vi "关键参数交互.vi"(9 "量程选择":enum16{"低量程", "高量程", "0-2量程"}(ring), 10 "测量模式(公式)":u16(ring)=1 items=["水样测试"=1, "标样核查"=2, "零点核查"=3, "跨度核查"=4, "空白测试"=5, "平行样"=6, "加标回收"=7], 11 "模型":enum32{"线性", "多项式"}(ring)) -> ()   [LabVIEW 2016]
panel:
  out "x != y?":T1
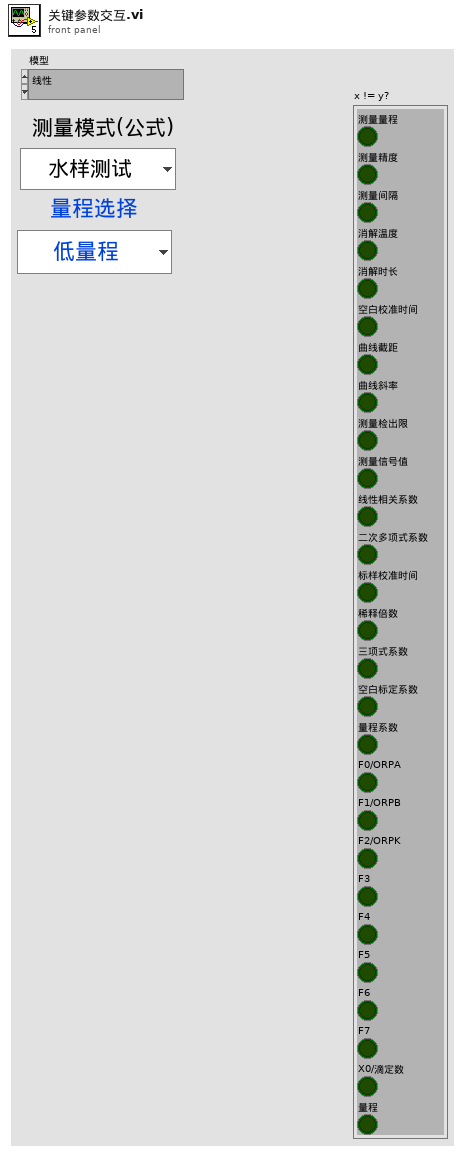
[diagram p1: front panel]
types:
  T1 = cluster{"测量量程":bool, "测量精度":bool, "测量间隔":bool, "消解温度":bool, "消解时长":bool, "空白校准时间":bool, "曲线截距":bool, "曲线斜率":bool, "测量检出限":bool, "测量信号值":bool, "线性相关系数":bool, "二次多项式系数":bool, "标样校准时间":bool, "稀释倍数":bool, "三项式系数":bool, "空白标定系数":bool, "量程系数":bool, "F0/ORPA":bool, "F1/ORPB":bool, "F2/ORPK":bool, "F3":bool, "F4":bool, "F5":bool, "F6":bool, "F7":bool, "X0/滴定数":bool, "量程":bool}
  T2 = cluster{"chose":string, "公式":cluster{"X^2":dbl, "X":dbl, "b":dbl}}
  T3 = cluster{"测量量程":dbl, "测量精度":dbl, "测量间隔":dbl, "消解温度":dbl, "消解时长":dbl, "空白校准时间":timestamp, "曲线截距":dbl, "曲线斜率":dbl, "测量检出限":dbl, "测量信号值":dbl, "线性相关系数":dbl, "二次多项式系数":dbl, "标样校准时间":timestamp, "稀释倍数":dbl, "三项式系数":dbl, "空白标定系数":dbl, "量程系数":dbl, "F0/ORPA":dbl, "F1/ORPB":dbl, "F2/ORPK":dbl, "F3":dbl, "F4":dbl, "F5":dbl, "F6":dbl, "F7":dbl, "X0/滴定数":dbl, "量程":dbl}
  T4 = cluster{"时间标识":timestamp, "设备":string, "日志信息":string, "流程参数":string}
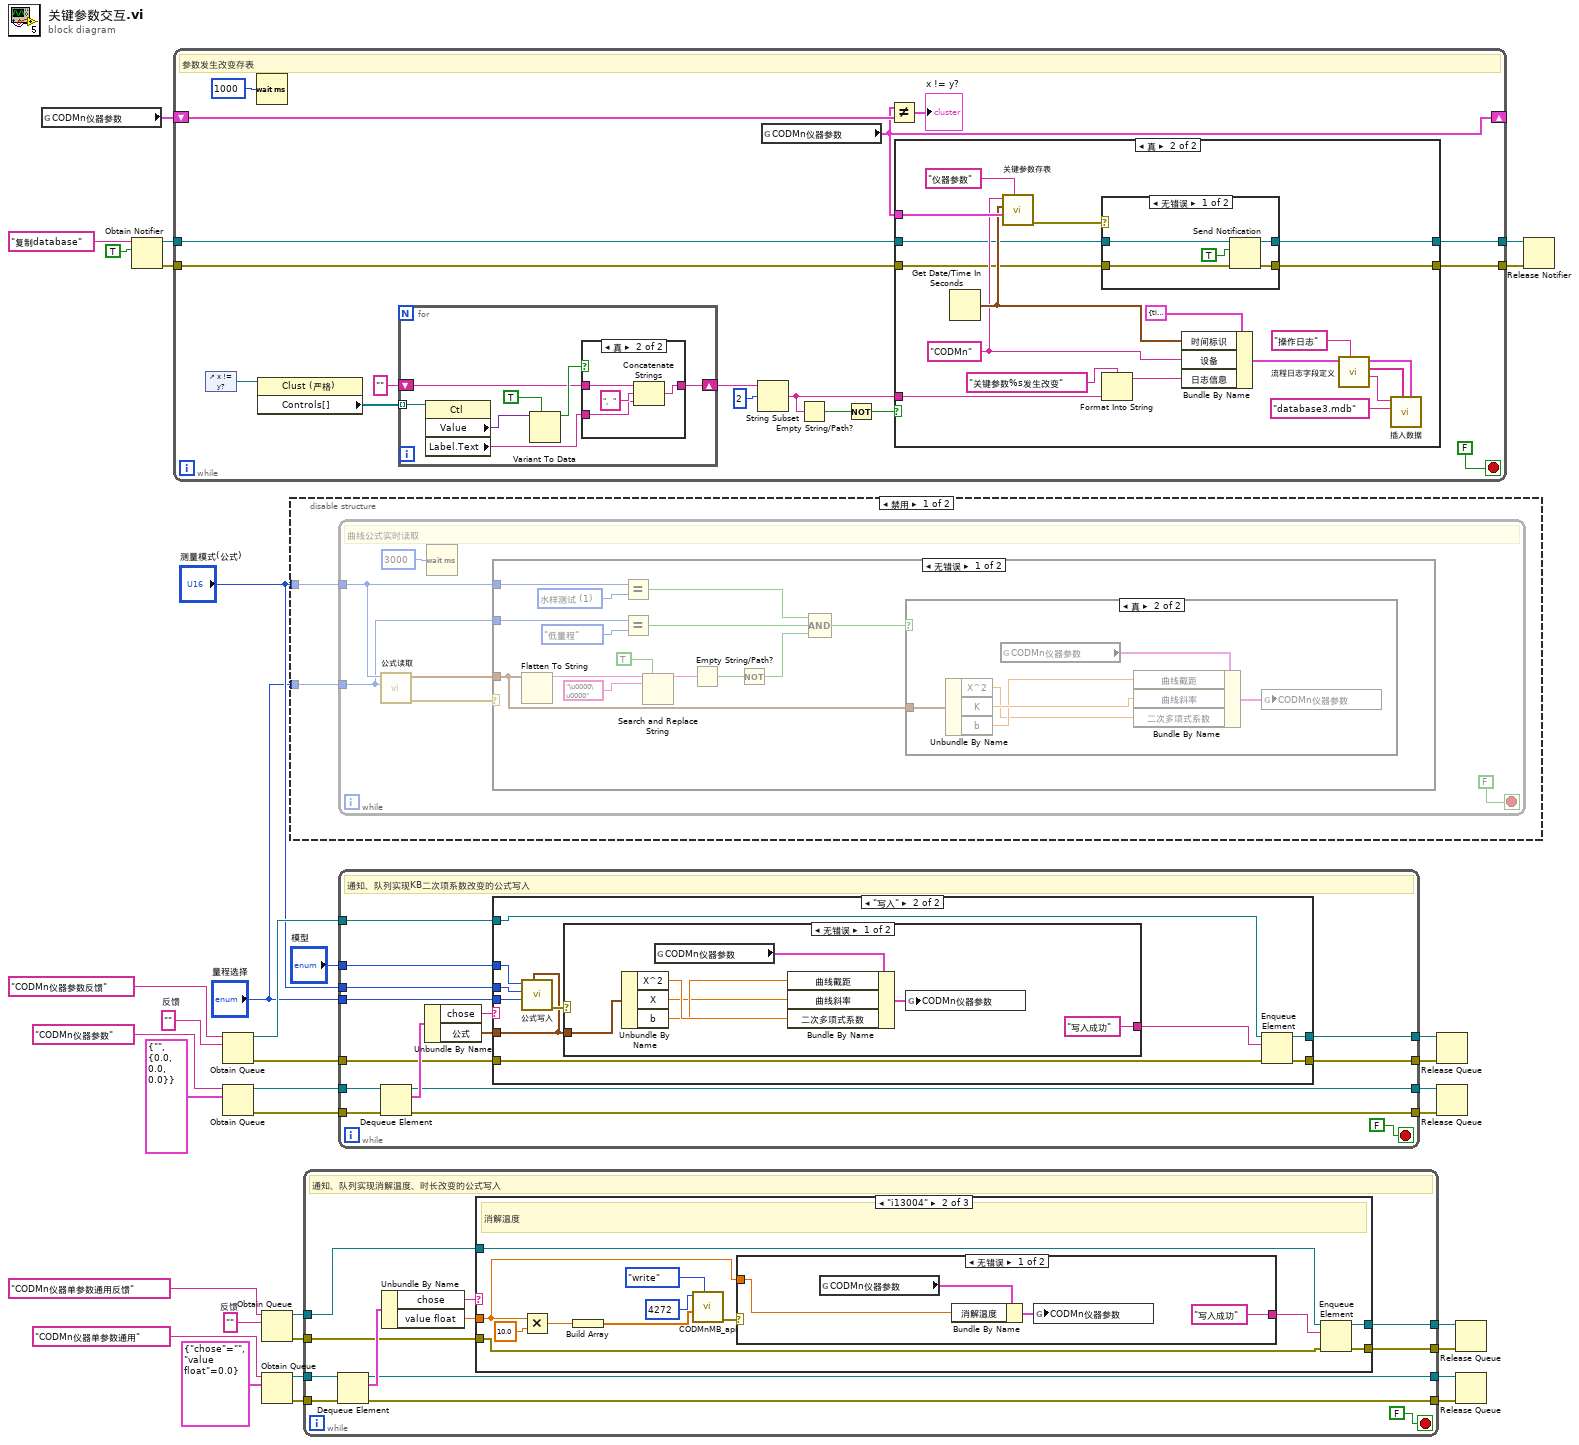
[diagram p0: block diagram]
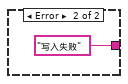
[diagram p6: hidden frame]
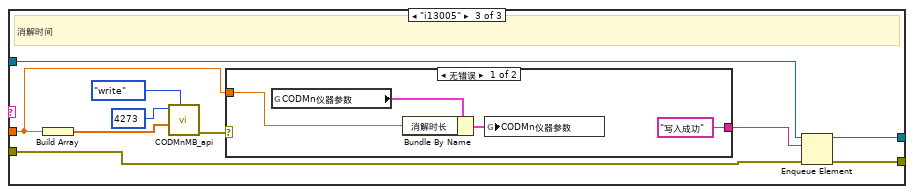
[diagram p7: hidden frame]
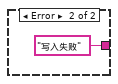
[diagram p8: hidden frame]
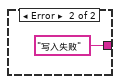
[diagram p10: hidden frame]
diagram:
  w9 = ""  # 反馈
  w25 = ""  # 反馈
  n1 = global read "CODMn断电保存全局变量.vi" "CODMn仪器参数"() -> (w34:T3)
  n2 = Obtain Notifier(name (unnamed)="复制database" ("名称（未命名）"), notification data type=TRUE) -> (notifier out=w19:refnum<notifier>, error out=w18:errorcluster)  [unwired: 2 in, 1 out]
  n3 = while {
    shift-right: [w46] -> _
    shift-left: w34 -> [w49]
    tunnel: w19 -> [w42]
    tunnel: w18 -> [w45]
    tunnel: [w44] -> w17
    tunnel: [w43] -> w16
    stop <- FALSE stop-if-true
    # "参数发生改变存表"
    n4 = control-ref of="x != y?"() -> (w47:refnum<vi>)
    n5 = Wait (ms)(milliseconds to wait=u32 1000 ("等待时间（毫秒）")) -> ()  [unwired: 1 out]
    n6 = property class="Clust (严格)"(reference=w47) -> ("Controls[]"=w37:refnum<vi>[])  [unwired: 1 in, 2 out]
    n7 = for {
      tunnel: w37 -> [w58] mode=indexing
      shift-right: [w52] -> w39
      shift-left: "" -> [w54]
      n8 = property class="Ctl"(reference=w58) -> ("Value"=w56:variant, "Label.Text"=w53:string)  [unwired: 1 in, 2 out]
      n9 = Variant To Data(type=TRUE, Variant=w56) -> (data=w55:bool)  [unwired: 1 in, 1 out]
      n10 = case shown="真" w55 {
        tunnel: w54 -> [w59 w63]
        tunnel: w53 -> [_ w60]
        tunnel: [w59 w62] -> w52
        frame False {
        }
        frame True {
          n11 = Concatenate Strings(w63, "、", w60) -> (w62:string)
        }
      }
    }
    n12 = String Subset(string=w39, offset (0)=2 ("偏移量(0)")) -> (substring=w35:string)  [unwired: 1 in]
    n13 = global read "CODMn断电保存全局变量.vi" "CODMn仪器参数"() -> (w46:T3)
    n14 = Empty String/Path?(string/path=w35) -> (empty?=w41:bool)
    n15 = Not(x=w41) -> (.not. x?=w36:bool)
    n16 = Not Equal?(x=w46, y=w49) -> (x != y?=→"x != y?":T1)
    n17 = case shown="真" w36 {
      tunnel: w46 -> [_ w83]
      tunnel: w35 -> [_ w78]
      tunnel: w45 -> [w65 w69]
      tunnel: [w64 w68] -> w44
      tunnel: [w65 w67] -> w43
      tunnel: w42 -> [w64 w66]
      frame False {
      }
      frame True {
        w80 = "CODMn" ("仪器名称")
        n18 = Get Date/Time In Seconds() -> (seconds since 1Jan1904=w81:timestamp)
        n19 = call "关键参数存表.vi"("table"="仪器参数", "仪器参数"=w83, "datatime"=w81, "仪器名称"=w80) -> ("error out"=w70:errorcluster)  [unwired: 7 in]
        n20 = case shown="无错误" w70 {
          tunnel: w66 -> [w89 w91]
          tunnel: w69 -> [w88 w90]
          tunnel: [w86 w91] -> w68
          tunnel: [w85 w90] -> w67
          frame No Error {
            n21 = Send Notification(notification=TRUE ("通知"), notifier=w89, error in (no error)=w88) -> (notifier out=w86:refnum<notifier>, error out=w85:errorcluster)
          }
          frame Error {
          }
        }
        n22 = Format Into String(format string="关键参数%s发生改变" ("格式字符串"), w78) -> (resulting string=w77:string)  [unwired: 2 in, 1 out]
        n23 = Bundle By Name(cluster=T4 {"时间标识"=timestamp(0 s since 1904-01-01), "设备"="", "日志信息"="", "流程参数"=""} ("data in"), "时间标识"=w81, "设备"=w80, "日志信息"=w77) -> (w71:T4)
        n24 = call "流程日志字段定义.vi"("table输入"="操作日志", "data in"=w71) -> ("table输出"=w74:string, "columns"=w75:string[], "data out"=w76:T4)  [unwired: 7 in]
        n25 = call "插入数据.vi"("data"=w76, "columns"=w75, "database"="database3.mdb", "table"=w74) -> ()  [unwired: 7 in, 1 out]
      }
    }
  }
  n26 = Obtain Queue(name (unnamed)="CODMn仪器参数反馈" ("名称（未命名）"), element data type=w25) -> (queue out=w26:refnum<queue>, error out=w24:errorcluster)  [unwired: 3 in, 1 out]
  n27 = Obtain Queue(name (unnamed)="CODMn仪器参数" ("名称（未命名）"), element data type=T2 {"chose"="", "公式"={"X^2"=0.0, "X"=0.0, "b"=0.0}}) -> (queue out=w33:refnum<queue>, error out=w32:errorcluster)  [unwired: 3 in, 1 out]
  n28 = Obtain Queue(name (unnamed)="CODMn仪器单参数通用反馈" ("名称（未命名）"), element data type=w9) -> (queue out=w8:refnum<queue>, error out=w10:errorcluster)  [unwired: 3 in, 1 out]
  n29 = Obtain Queue(name (unnamed)="CODMn仪器单参数通用" ("名称（未命名）"), element data type=cluster{"chose":string, "value float":dbl} {"chose"="", "value float"=0.0}) -> (queue out=w1:refnum<queue>, error out=w2:errorcluster)  [unwired: 3 in, 1 out]
  n30 = disable-structure shown="禁用" {
    disable-tunnel: "测量模式(公式)" -> [w93 _]
    disable-tunnel: "量程选择" -> [w92 _]
    frame Disabled {
      n31 = while {
        tunnel: w93 -> [w96]
        tunnel: w92 -> [w95]
        stop <- FALSE stop-if-true
        # "曲线公式实时读取"
        n32 = call "公式读取.vi"("量程选择"=w95, "测量模式(公式)"=w96) -> ("error out"=w94:errorcluster, "方程系数"=w97:cluster{"K":dbl, "b":dbl, "X^2":dbl})  [unwired: 8 in]
        n33 = Wait (ms)(milliseconds to wait=u32 3000 ("等待时间（毫秒）")) -> ()  [unwired: 1 out]
        n34 = case shown="无错误" w94 {
          tunnel: w96 -> [w113 _]
          tunnel: w97 -> [w103 _]
          tunnel: w95 -> [w109 _]
          frame No Error {
            w108 = u16 1 items=["水样测试"=1, "标样核查"=2, "零点核查"=3, "跨度核查"=4, "空白测试"=5, "平行样"=6, "加标回收"=7] ("测量模式(公式)")
            n35 = Flatten To String(anything=w103) -> (data string=w106:string)  [unwired: 3 in, 2 out]
            n36 = Equal?(x=w113, y=w108) -> (x = y?=w112:bool)
            n37 = Equal?(x=w109, y=enum16{"低量程", "高量程", "0-2量程"}."低量程" ("量程选择")) -> (x = y?=w111:bool)
            n38 = Search and Replace String(replace all?=TRUE ("替换全部？(F)"), input string=w106, search string="\u0000\u0000" ("数据字符串")) -> (result string=w102:string)  [unwired: 5 in, 3 out]
            n39 = Empty String/Path?(string/path=w102) -> (empty?=w101:bool)
            n40 = Not(x=w101) -> (.not. x?=w100:bool)
            n41 = Compound Arithmetic op=AND ("复合运算")(w112, w111, w100) -> (w110:bool)
            n42 = case shown="真" w110 {
              tunnel: w103 -> [_ w119]
              frame False {
              }
              frame True {
                n43 = Unbundle By Name(w119) -> ("X^2"=w116:dbl, "K"=w118:dbl, "b"=w117:dbl)
                n44 = global read "CODMn断电保存全局变量.vi" "CODMn仪器参数"() -> (w115:T3)
                n45 = Bundle By Name(cluster=w115, "曲线截距"=w117, "曲线斜率"=w118, "二次多项式系数"=w116) -> (w114:T3)
                n46 = global write "CODMn断电保存全局变量.vi" "CODMn仪器参数"(w114) -> ()
              }
            }
          }
          frame Error {
          }
        }
      }
    }
    frame Enabled {
    }
  }
  n47 = while {
    tunnel: w1 -> [w130]
    tunnel: w2 -> [w129]
    tunnel: [w125] -> w5
    tunnel: [w124] -> w6
    tunnel: w8 -> [w123]
    tunnel: w10 -> [w122]
    tunnel: [w121] -> w11
    tunnel: [w120] -> w12
    stop <- FALSE stop-if-true
    # "通知、队列实现消解温度、时长改变的公式写入"
    n48 = Dequeue Element(queue=w130, error in (no error)=w129) -> (queue out=w125:refnum<queue>, element=w128:cluster{"chose":string, "value float":dbl}, error out=w124:errorcluster)  [unwired: 1 in, 1 out]
    n49 = Unbundle By Name(w128) -> ("chose"=w127:string, "value float"=w126:dbl)
    n50 = case shown="\"i13004\"" w127 {
      tunnel: w126 -> [_ w134 w151]
      tunnel: w123 -> [w133 w145 w160]
      tunnel: w122 -> [w132 w143 w156]
      tunnel: [w133 w142 w158] -> w121
      tunnel: [w132 w141 w157] -> w120
      frame "假", Default {
      }
      frame "i13004" {
        # "消解温度"
        n51 = Multiply(x=w134, y=10.0) -> (x*y=w137:dbl)
        n52 = Build Array(w137) -> (w136:dbl[])
        n53 = call "CODMnMB_api.vi"("STEP"=enum16{"open", "read", "write", "close"}."write", "values"=w136, "starting address"=u16 4272) -> ("error out"=w135:errorcluster)  [unwired: 6 in, 2 out]
        n54 = case shown="无错误" w135 {
          tunnel: ["写入成功" ("消息") "写入失败" ("消息")] -> w144
          tunnel: w134 -> [w146 _]
          frame No Error {
            n55 = global read "CODMn断电保存全局变量.vi" "CODMn仪器参数"() -> (w148:T3)
            n56 = Bundle By Name(cluster=w148, "消解温度"=w146) -> (w147:T3)
            n57 = global write "CODMn断电保存全局变量.vi" "CODMn仪器参数"(w147) -> ()
          }
          frame Error {
          }
        }
        n58 = Enqueue Element(queue=w145, element=w144, error in (no error)=w143) -> (queue out=w142:refnum<queue>, error out=w141:errorcluster)  [unwired: 1 in, 1 out]
      }
      frame "i13005" {
        # "消解时间"
        n59 = Build Array(w151) -> (w153:dbl[])
        n60 = call "CODMnMB_api.vi"("STEP"=enum16{"open", "read", "write", "close"}."write", "values"=w153, "starting address"=u16 4273) -> ("error out"=w152:errorcluster)  [unwired: 6 in, 2 out]
        n61 = case shown="无错误" w152 {
          tunnel: ["写入成功" ("消息") "写入失败" ("消息")] -> w159
          tunnel: w151 -> [w162 _]
          frame No Error {
            n62 = global read "CODMn断电保存全局变量.vi" "CODMn仪器参数"() -> (w163:T3)
            n63 = Bundle By Name(cluster=w163, "消解时长"=w162) -> (w161:T3)
            n64 = global write "CODMn断电保存全局变量.vi" "CODMn仪器参数"(w161) -> ()
          }
          frame Error {
          }
        }
        n65 = Enqueue Element(queue=w160, element=w159, error in (no error)=w156) -> (queue out=w158:refnum<queue>, error out=w157:errorcluster)  [unwired: 1 in, 1 out]
      }
    }
  }
  n66 = while {
    tunnel: w33 -> [w179]
    tunnel: w32 -> [w178]
    tunnel: [w174] -> w29
    tunnel: [w173] -> w28
    tunnel: w26 -> [w172]
    tunnel: w24 -> [w171]
    tunnel: [w170] -> w23
    tunnel: [w169] -> w22
    tunnel: "模型" -> [w168]
    tunnel: "测量模式(公式)" -> [w167]
    tunnel: "量程选择" -> [w166]
    stop <- FALSE stop-if-true
    # "通知、队列实现KB二次项系数改变的公式写入"
    n67 = Dequeue Element(queue=w179, error in (no error)=w178) -> (queue out=w174:refnum<queue>, element=w177:T2, error out=w173:errorcluster)  [unwired: 1 in, 1 out]
    n68 = Unbundle By Name(w177) -> ("chose"=w176:string, "公式"=w175:cluster{"X^2":dbl, "X":dbl, "b":dbl})
    n69 = case shown="\"写入\"" w176 {
      tunnel: w175 -> [_ w183]
      tunnel: w172 -> [w182 w192]
      tunnel: w171 -> [w181 w190]
      tunnel: [w182 w189] -> w170
      tunnel: [w181 w188] -> w169
      tunnel: w168 -> [_ w186]
      tunnel: w167 -> [_ w185]
      tunnel: w166 -> [_ w184]
      frame "假", Default {
      }
      frame "写入" {
        n70 = call "公式写入.vi"("公式"=w183, "量程选择"=w184, "测量模式(公式)"=w185, "模型"=w186) -> ("error out"=w187:errorcluster)  [unwired: 7 in]
        n71 = case shown="无错误" w187 {
          tunnel: ["写入成功" ("消息") "写入失败" ("消息")] -> w191
          tunnel: w183 -> [w193 _]
          frame No Error {
            n72 = Unbundle By Name(w193) -> ("X^2"=w196:dbl, "X"=w194:dbl, "b"=w195:dbl)
            n73 = global read "CODMn断电保存全局变量.vi" "CODMn仪器参数"() -> (w197:T3)
            n74 = Bundle By Name(cluster=w197, "曲线截距"=w195, "曲线斜率"=w194, "二次多项式系数"=w196) -> (w198:T3)
            n75 = global write "CODMn断电保存全局变量.vi" "CODMn仪器参数"(w198) -> ()
          }
          frame Error {
          }
        }
        n76 = Enqueue Element(queue=w192, element=w191, error in (no error)=w190) -> (queue out=w189:refnum<queue>, error out=w188:errorcluster)  [unwired: 1 in, 1 out]
      }
    }
  }
  n77 = Release Queue(queue=w23, error in (no error)=w22) -> ()  [unwired: 1 in, 3 out]
  n78 = Release Queue(queue=w29, error in (no error)=w28) -> ()  [unwired: 1 in, 3 out]
  n79 = Release Queue(queue=w11, error in (no error)=w12) -> ()  [unwired: 1 in, 3 out]
  n80 = Release Queue(queue=w5, error in (no error)=w6) -> ()  [unwired: 1 in, 3 out]
  n81 = Release Notifier(notifier=w17, error in (no error)=w16) -> ()  [unwired: 1 in, 3 out]
